vi "Winchton.vi"(10 "Auto Drive Button":bool) -> ()   [LabVIEW 2016]
uses:
  AutoaimVar.vi
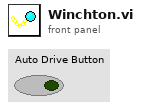
[diagram p1: front panel]
types:
  T1 = typedef "WPI_MotorControlDeviceRef.ctl" = cluster{"DeviceStatus":errorcluster, "Type":T2, "PWM":cluster{"PWM Channel":T3, "DeadBand":T4}, "CAN":cluster{"Device Number":u8, "SetOutput VI Ref":variant, "GetOutput VI Ref":variant, "Enable VI Ref":variant, "Disable VI Ref":variant, "Data":variant}, "Invert":bool}
  T2 = typedef "WPI_MotorControlType.ctl" = enum16{"PWM", "CAN"}
  T3 = typedef "FPGA_DIOPWMChannel.ctl" = enum8{"PWM 0", "PWM 1", "PWM 2", "PWM 3", "PWM 4", "PWM 5", "PWM 6", "PWM 7", "PWM 8", "PWM 9", "PWM MXP 0", "PWM MXP 1", "PWM MXP 2", "PWM MXP 3", "PWM MXP 4", "PWM MXP 5", "PWM MXP 6", "PWM MXP 7", "PWM MXP 8", "PWM MXP 9", "Invalid"}
  T4 = typedef "WPI_PWMDeadband.ctl" = cluster{"Name":string, "maxPositivePwm":i32, "minPositivePwm":i32, "centerPwm":i32, "maxNegativePwm":i32, "minNegativePwm":i32, "angularRange":u16}
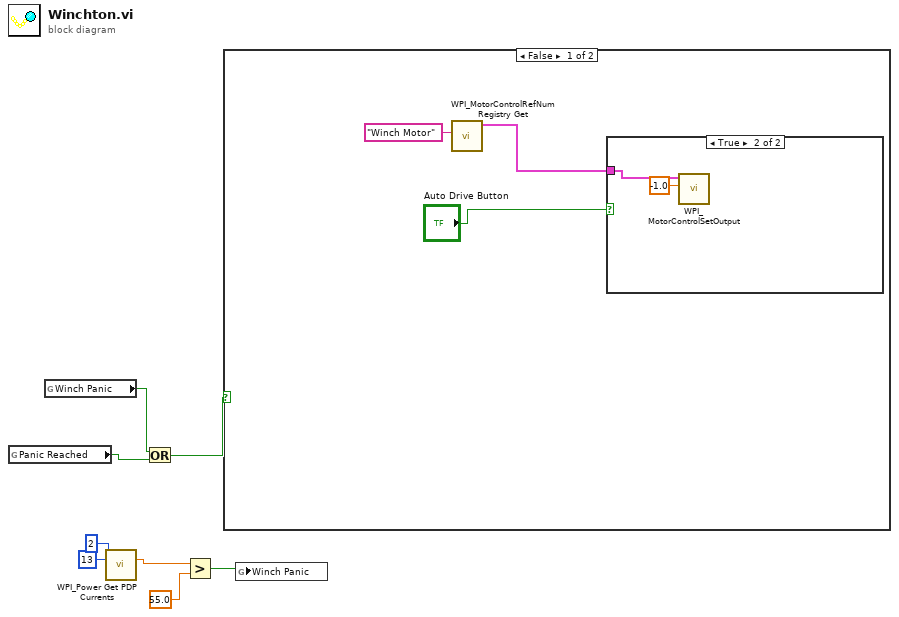
[diagram p0: block diagram]
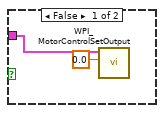
[diagram p2: hidden frame]
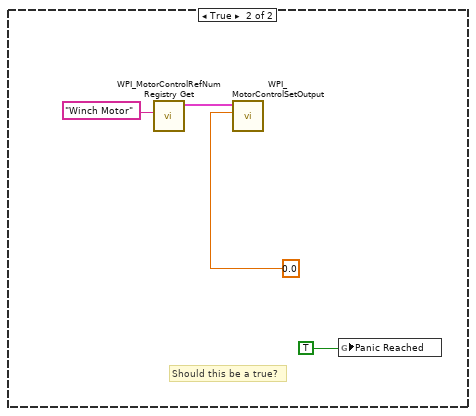
[diagram p3: hidden frame]
diagram:
  n1 = global read "AutoaimVar.vi" "Panic Reached"() -> (w8:bool)
  n2 = global read "AutoaimVar.vi" "Winch Panic"() -> (w7:bool)
  n3 = call <vilib>:"WPI_Power Get PDP Currents.vi"("Power Distribution Panel (0)"=u8 2, "PDP Channel"=13) -> ("current (A)"=w3:dbl)  [unwired: 11 in, 2 out]
  n4 = Or(x=w7, y=w8) -> (x .or. y?=w6:bool)
  n5 = Greater?(x=w3, y=55.0) -> (0:w1:bool)
  n6 = case shown="False" w6 {
    frame False {
      n7 = call <vilib>:"WPI_MotorControlRefNum Registry Get.vi"("refnum name"="Winch Motor") -> ("MotorControlDevRef"=w9:T1)  [unwired: 9 in, 1 out]
      n8 = case shown="True" "Auto Drive Button" {
        tunnel: w9 -> [w13 w15]
        frame False {
          n9 = call <vilib>:"WPI_MotorControlSetOutput.vi"("Output"=0.0, "MotorControlDevRef"=w13) -> ()  [unwired: 7 in, 3 out]
        }
        frame True {
          n10 = call <vilib>:"WPI_MotorControlSetOutput.vi"("Output"=-1.0, "MotorControlDevRef"=w15) -> ()  [unwired: 7 in, 3 out]
        }
      }
    }
    frame True {
      # "Should this be a true?"
      n11 = call <vilib>:"WPI_MotorControlRefNum Registry Get.vi"("refnum name"="Winch Motor") -> ("MotorControlDevRef"=w16:T1)  [unwired: 9 in, 1 out]
      n12 = call <vilib>:"WPI_MotorControlSetOutput.vi"("Output"=0.0, "MotorControlDevRef"=w16) -> ()  [unwired: 7 in, 3 out]
      n13 = global write "AutoaimVar.vi" "Panic Reached"(TRUE) -> ()
    }
  }
  n14 = global write "AutoaimVar.vi" "Winch Panic"(w1) -> ()
